vi "wait.vi"(8 "error in (no error)":errorcluster, 10 "Wait ms":u32, 11 "Model in":refnum<class "Model.lvclass">) -> (0 "error out":errorcluster, 3 "Model out":refnum<class "Model.lvclass">)   [LabVIEW 2015]
uses:
  Model.lvclass
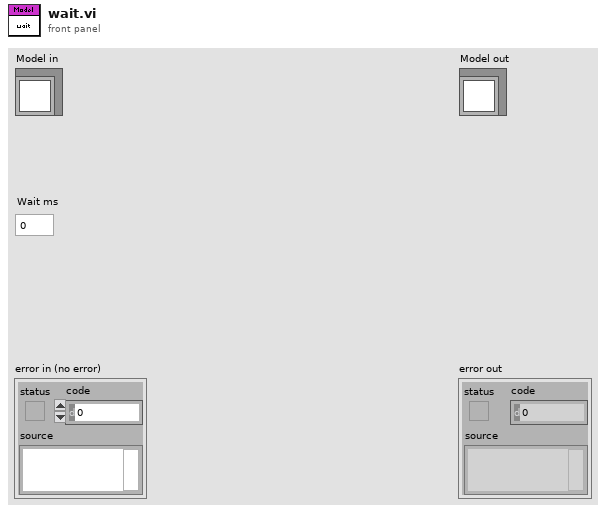
[diagram p1: front panel]
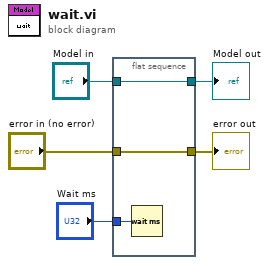
[diagram p0: block diagram]
diagram:
  n1 = flat-sequence {
    tunnel: "error in (no error)" -> [w8]
    tunnel: [w8] -> w4
    tunnel: [w7] -> w3
    tunnel: "Model in" -> [w7]
    tunnel: "Wait ms" -> [w6]
    frame #0 {
      n2 = Wait (ms)(milliseconds to wait=w6) -> ()  [unwired: 1 out]
    }
  }
  "error out" <- w4
  "Model out" <- w3
